vi "Describe Comparison.vi"(6 "Equal?":bool, 8 "error in (no error)":errorcluster, 9 "Control Value 2":variant, 10 "Control Value 1":variant) -> (0 "error out":errorcluster, 2 "Description":string)   [LabVIEW 2020, in "Identical Inputs Comparator.lvclass"]
uses:
  Identical Inputs Comparator.lvclass
  Core/Comparator/Comparator.lvclass
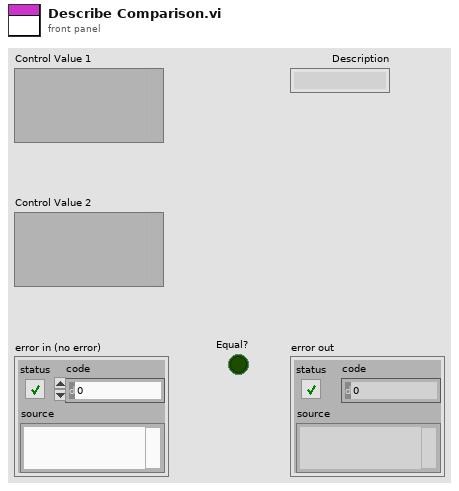
[diagram p1: front panel]
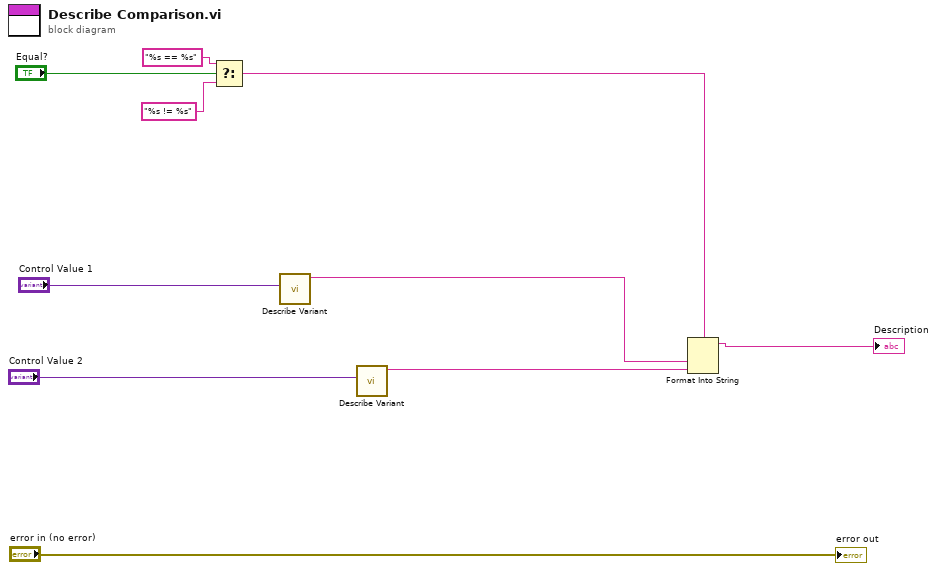
[diagram p0: block diagram]
diagram:
  n1 = Select(t="%s == %s", s="Equal?", f="%s != %s") -> (s? t:f=w6:string)
  n2 = call "Describe Variant.vi"("Variant"="Control Value 1") -> ("Description with Type"=w2:string)  [unwired: 8 in, 2 out]
  n3 = call "Describe Variant.vi"("Variant"="Control Value 2") -> ("Description with Type"=w1:string)  [unwired: 8 in, 2 out]
  n4 = Format Into String(format string=w6, w2, w1) -> (resulting string=→"Description":string)  [unwired: 2 in, 1 out]
  "error out" <- "error in (no error)"
